vi "HW2_陣列排列組合.vi"() -> ()   [LabVIEW 2018]
panel:
  out "by N (0為不屬於任何類型)":dbl[](array[numeric])
  out "high/lower peak":dbl[][](array[numeric])
  out "斜率":dbl[][](array[numeric])
  out "Array":i32[](array[numeric])
  out "有n!組排列組合":i32[](array[numeric])
  out "排列組合":i32[][](array[numeric])
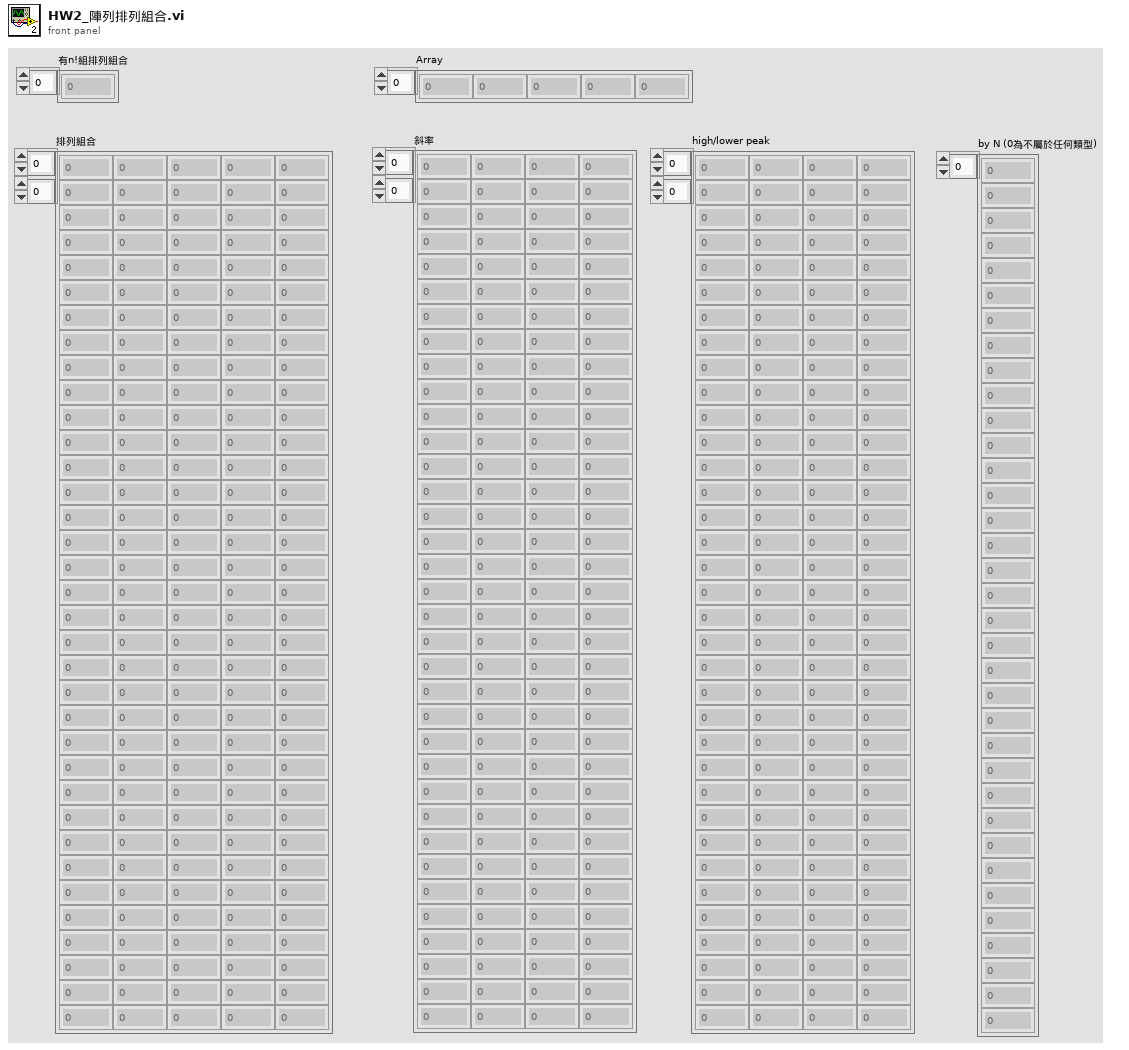
[diagram p1: front panel]
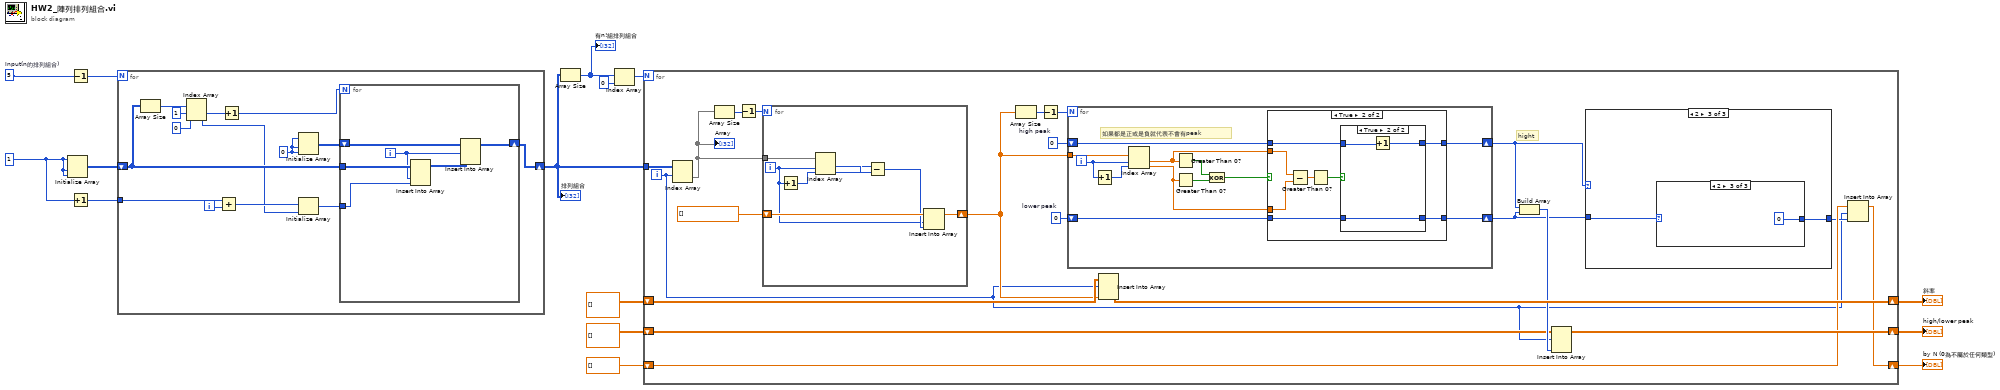
[diagram p0: block diagram]
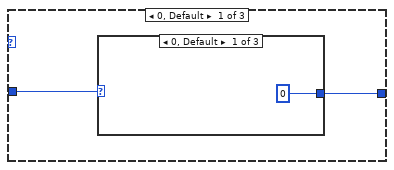
[diagram p2: hidden frame]
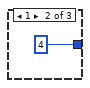
[diagram p3: hidden frame]
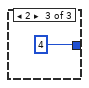
[diagram p4: hidden frame]
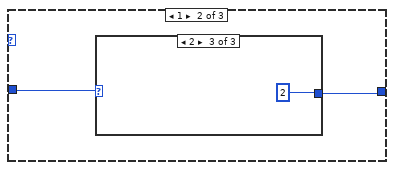
[diagram p5: hidden frame]
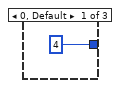
[diagram p6: hidden frame]
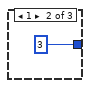
[diagram p7: hidden frame]
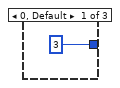
[diagram p8: hidden frame]
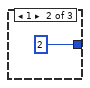
[diagram p9: hidden frame]
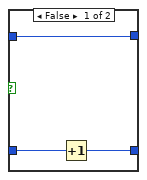
[diagram p11: hidden frame]
diagram:
  w7 = 5  # Input(n的排列組合)
  w8 = 1
  n1 = Initialize Array(w8, w8, w8) -> (w14:i32[][])
  n2 = Decrement(x=w7) -> (x-1=w15:i32)
  n3 = Increment(x=w8) -> (x+1=w13:i32)
  n4 = for {
    N: w15 -> [_]
    tunnel: w13 -> [w21]
    shift-right: [w17] -> w9
    shift-left: w14 -> [w22]
    i -> [w16]
    w23 = 0 ("dimension size")
    n5 = Array Size(array=w22) -> (size(s)=w28:i32[])
    n6 = Index Array(array=w28, index #1=1 ("index (row)"), index #2=0 ("disabled index (col)")) -> (element #1=w26:i32, element #2=w19:i32)
    n7 = Add(x=w21, y=w16) -> (x+y=w20:i32)
    n8 = Increment(x=w26) -> (x+1=w25:i32)
    n9 = Initialize Array(w23, w23, w23) -> (w24:i32[][])
    n10 = Initialize Array(w20, w19) -> (w18:i32[])
    n11 = for {
      N: w25 -> [_]
      tunnel: w22 -> [w33]
      shift-right: [w35] -> w17
      shift-left: w24 -> [w34]
      tunnel: w18 -> [w32]
      i -> [w31]
      n12 = Insert Into Array(array=w33, index (col)=w31, new element=w32) -> (w30:i32[][])  [unwired: 1 in]
      n13 = Insert Into Array(array=w34, index (row)=w31, new element=w30) -> (w35:i32[][])  [unwired: 1 in]
    }
  }
  "排列組合" <- w9
  n14 = Array Size(array=w9) -> (size(s)=w12:i32[])
  "有n!組排列組合" <- w12
  n15 = Index Array(array=w12, index=0) -> (element=w10:i32)
  n16 = for {
    N: w10 -> [_]
    tunnel: w9 -> [w56]
    shift-right: [w50] -> w5
    shift-left: dbl[][] [] -> [w51]
    shift-right: [w42] -> w3
    shift-left: dbl[][] [] -> [w43]
    shift-right: [w36] -> w1
    shift-left: dbl[] [] -> [w39]
    i -> [w37]
    w45 = 0  # lower peak
    w46 = 0  # high peak
    # "hight"
    n17 = Index Array(array=w56, index (row)=w37) -> (element=w55:i32[])  [unwired: 1 in]
    "Array" <- w55
    n18 = Array Size(array=w55) -> (size(s)=w52:i32)
    n19 = Decrement(x=w52) -> (x-1=w54:i32)
    n20 = for {
      N: w54 -> [_]
      tunnel: w55 -> [w107]
      shift-right: [w101] -> w47
      shift-left: dbl[] [] -> [w105]
      i -> [w100]
      n21 = Increment(x=w100) -> (x+1=w106:i32)
      n22 = Index Array(array=w107, index #1=w100, index #2=w106) -> (element #1=w104:i32, element #2=w103:i32)
      n23 = Subtract(x=w103, y=w104) -> (x-y=w102:i32)
      n24 = Insert Into Array(array=w105, index=w100, new element=w102) -> (w101:dbl[])
    }
    n25 = Array Size(array=w47) -> (size(s)=w49:i32)
    n26 = Decrement(x=w49) -> (x-1=w48:i32)
    n27 = for {
      N: w48 -> [_]
      tunnel: w47 -> [w81]
      shift-right: [w77] -> w41
      shift-left: w46 -> [w80]
      shift-right: [w78] -> w40
      shift-left: w45 -> [w79]
      i -> [w82]
      # "如果都是正或是負就代表不會有peak"
      n28 = Increment(x=w82) -> (x+1=w83:i32)
      n29 = Index Array(array=w81, index #1=w82, index #2=w83) -> (element #1=w75:dbl, element #2=w74:dbl)
      n30 = Greater Than 0?(x=w75) -> (x > 0?=w76:bool)
      n31 = Greater Than 0?(x=w74) -> (x > 0?=w72:bool)
      n32 = Exclusive Or(1:w72, 2:w76) -> (0:w73:bool)
      n33 = case shown="True" w73 {
        tunnel: w80 -> [w85 w91]
        tunnel: w79 -> [w84 w90]
        tunnel: [w84 w89] -> w78
        tunnel: [w85 w88] -> w77
        tunnel: w75 -> [_ w86]
        tunnel: w74 -> [_ w87]
        frame False {
        }
        frame True {
          n34 = Subtract(x=w86, y=w87) -> (x-y=w92:dbl)
          n35 = Greater Than 0?(x=w92) -> (x > 0?=w93:bool)
          n36 = case shown="True" w93 {
            tunnel: w91 -> [w96 w99]
            tunnel: w90 -> [w95 w98]
            tunnel: [w96 w97] -> w88
            tunnel: [w94 w98] -> w89
            frame False {
              n37 = Increment(x=w95) -> (x+1=w94:i32)
            }
            frame True {
              n38 = Increment(x=w99) -> (x+1=w97:i32)
            }
          }
        }
      }
    }
    n39 = Insert Into Array(array=w51, index (row)=w37, new element=w47) -> (w50:dbl[][])  [unwired: 1 in]
    n40 = Build Array(w41, w40) -> (w44:i32[])
    n41 = Insert Into Array(array=w43, index (row)=w37, new element=w44) -> (w42:dbl[][])  [unwired: 1 in]
    n42 = case shown="2" w41 {
      tunnel: w40 -> [w57 w63 w67]
      tunnel: [w58 w62 w68] -> w38
      frame 0, Default {
        n43 = case shown="0, Default" w57 {
          tunnel: [0 ("y") 4 ("y") 4 ("y")] -> w58
          frame 0, Default {
          }
          frame 1 {
          }
          frame 2 {
          }
        }
      }
      frame 1 {
        n44 = case shown="2" w63 {
          tunnel: [4 ("y") 3 ("y") 2 ("y")] -> w62
          frame 0, Default {
          }
          frame 1 {
          }
          frame 2 {
          }
        }
      }
      frame 2 {
        n45 = case shown="2" w67 {
          tunnel: [3 ("y") 2 ("y") 0 ("y")] -> w68
          frame 0, Default {
          }
          frame 1 {
          }
          frame 2 {
          }
        }
      }
    }
    n46 = Insert Into Array(array=w39, index=w37, new element=w38) -> (w36:dbl[])
  }
  "斜率" <- w5
  "high/lower peak" <- w3
  "by N (0為不屬於任何類型)" <- w1
